vi "serial cmd-response.vi"(0 "VISA In":refnum<visa-resource-name>, 1 "mode":enum16{"wr & rd", "write", "read"}(ring), 3 "flush transcvr(F)":bool, 5 "cmd":string, 9 "ReadWait":u32=50, 11 "error in":errorcluster, 12 "Sem Timeout (5000)":i32=5000) -> (4 "VISA out":refnum<visa-resource-name>, 6 "rsp str out":string, 8 "cmd str out":string, 10 "timeout?":bool, 15 "error out":errorcluster)   [LabVIEW 2017]
doc: "Developed by: Kevin Thompson\nThompson Engineering\nthompson.engineering@comcast.net\n(510) 673-3614"
uses:
  <vilib>/Instr/_visa.llb/VISA Flush IO Buffer Mask.ctl
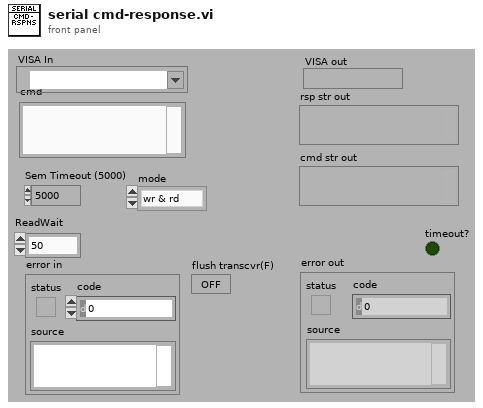
[diagram p1: front panel]
types:
  T1 = typedef "Semaphore RefNum" = refnum<k1>
  T2 = typedef "VISA Flush IO Buffer Mask.ctl" = u16
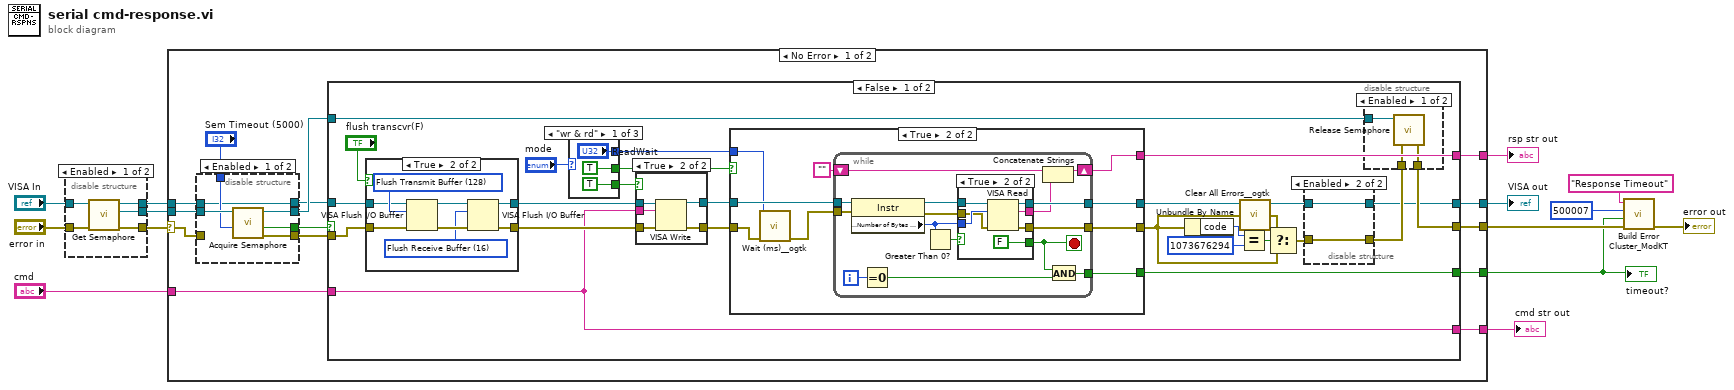
[diagram p0: block diagram]
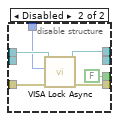
[diagram p3: hidden frame]
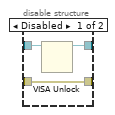
[diagram p4: hidden frame]
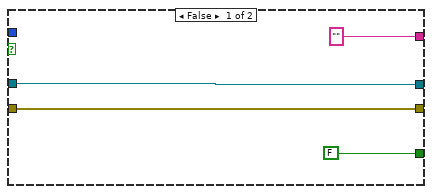
[diagram p7: hidden frame]
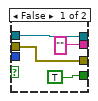
[diagram p8: hidden frame]
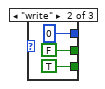
[diagram p10: hidden frame]
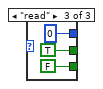
[diagram p11: hidden frame]
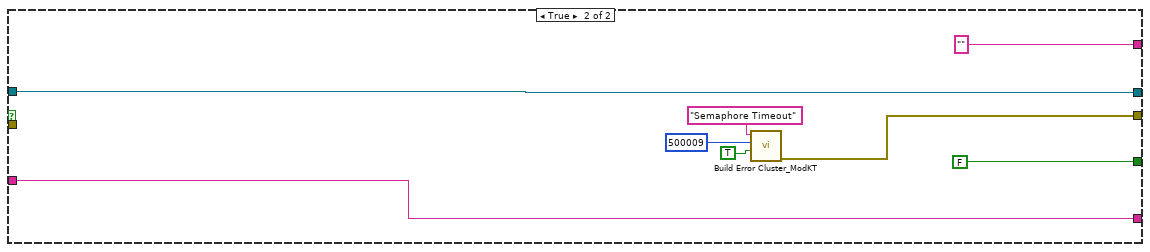
[diagram p12: hidden frame]
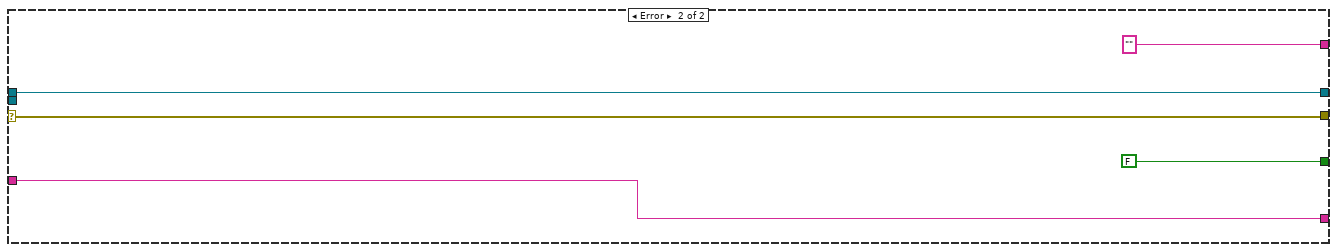
[diagram p13: hidden frame]
diagram:
  n1 = disable-structure shown="Enabled" {
    disable-tunnel: "VISA In" -> [w19 w21]
    disable-tunnel: "error in" -> [w18 w20]
    disable-tunnel: [w17 w21] -> w6
    disable-tunnel: [w16 w20] -> w5
    disable-tunnel: [w15 _] -> w4
    frame Enabled {
      n2 = call "Get Semaphore.vi"("error in"=w18, "VISA In"=w19) -> ("error out"=w16:errorcluster, "semaphore out"=w15:T1, "VISA Out"=w17:refnum<visa-resource-name>)  [unwired: 3 in]
    }
    frame Disabled {
    }
  }
  n3 = case shown="No Error" w5 {
    selector: w5 -> [w22 w156]
    tunnel: [w35 FALSE] -> w11
    tunnel: [w34 "" ("read buffer")] -> w14
    tunnel: w6 -> [w24 w157]
    tunnel: [w33 w157] -> w13
    tunnel: [w32 w156] -> w12
    tunnel: w4 -> [w31 _]
    tunnel: "cmd" -> [w26 w155]
    tunnel: [w25 w155] -> w2
    frame No Error {
      n4 = disable-structure shown="Enabled" {
        disable-tunnel: w31 -> [w41 _]
        disable-tunnel: "Sem Timeout (5000)" -> [w40 w42]
        disable-tunnel: [w39 FALSE ("timed out")] -> w29
        disable-tunnel: [w38 _] -> w28
        disable-tunnel: [w37 w47] -> w27
        disable-tunnel: w24 -> [w36 w46]
        disable-tunnel: [w36 w45] -> w23
        disable-tunnel: w22 -> [_ w44]
        frame Enabled {
          n5 = call <vilib>:"Acquire Semaphore.vi"("ms timeout (-1)"=w40, "semaphore"=w41) -> ("error out"=w37:errorcluster, "timed out"=w39:bool, "semaphore out"=w38:T1)  [unwired: 3 in]
        }
        frame Disabled {
          n6 = call <vilib>:"VISA Lock Async.vi"("error in (no error)"=w44, "timeout (0)"=w42, "VISA resource name"=w46) -> ("error out"=w47:errorcluster, "VISA resource name out"=w45:refnum<visa-resource-name>)  [unwired: 6 in, 1 out]
        }
      }
      n7 = case shown="False" w29 {
        tunnel: [w63 "" ("read buffer")] -> w34
        tunnel: [w62 FALSE] -> w35
        tunnel: w23 -> [w61 w152]
        tunnel: [w56 w149] -> w32
        tunnel: [w48 w152] -> w33
        tunnel: w28 -> [w57 _]
        tunnel: w27 -> [w55 _]
        tunnel: w26 -> [w54 w147]
        tunnel: [w54 w147] -> w25
        frame False {
          n8 = case shown="True" "flush transcvr(F)" {
            tunnel: w61 -> [w83 w90]
            tunnel: [w82 w87] -> w60
            tunnel: [w83 w86] -> w59
            tunnel: w55 -> [w82 w84]
            frame False {
            }
            frame True {
              w85 = T2 16 items=["Flush Receive Buffer"=16, "Write Transmit Buffer to Device"=32, "Flush Receive Buffer (No I/O)"=64, "Flush Transmit Buffer"=128] ("Mask")
              w91 = T2 128 items=["Flush Receive Buffer"=16, "Write Transmit Buffer to Device"=32, "Flush Receive Buffer (No I/O)"=64, "Flush Transmit Buffer"=128] ("Mask")
              n9 = VISA Flush I/O Buffer(VISA resource name=w90, mask (16)=w91, error in (no error)=w84) -> (VISA resource name out=w88:refnum<visa-resource-name>, error out=w89:errorcluster)
              n10 = VISA Flush I/O Buffer(VISA resource name=w88, mask (16)=w85, error in (no error)=w89) -> (VISA resource name out=w86:refnum<visa-resource-name>, error out=w87:errorcluster)
            }
          }
          n11 = case shown="\"wr & rd\"" "mode" {
            tunnel: [TRUE TRUE FALSE] -> w70
            tunnel: [TRUE FALSE TRUE] -> w69
            tunnel: ["ReadWait" u32 0 ("wait (ms)") u32 0 ("wait (ms)")] -> w53
            frame "wr & rd" {
            }
            frame "write" {
            }
            frame "read" {
            }
          }
          n12 = case shown="True" w70 {
            tunnel: [w132 w137] -> w72
            tunnel: [w131 w136] -> w52
            tunnel: w59 -> [w132 w135]
            tunnel: w54 -> [_ w134]
            tunnel: w60 -> [w131 w133]
            frame False {
            }
            frame True {
              n13 = VISA Write(VISA resource name=w135, write buffer=w134, error in (no error)=w133) -> (VISA resource name out=w137:refnum<visa-resource-name>, error out=w136:errorcluster)  [unwired: 1 out]
            }
          }
          n14 = case shown="True" w69 {
            tunnel: w72 -> [w93 w104]
            tunnel: [FALSE w100] -> w62
            tunnel: [w93 w103] -> w49
            tunnel: ["" ("read buffer") w99] -> w63
            tunnel: [w92 w102] -> w64
            tunnel: w53 -> [_ w98]
            tunnel: w52 -> [w92 w97]
            frame False {
            }
            frame True {
              n15 = call <userlib>:"Wait (ms)__ogtk.vi"("error in (no error)"=w97, "milliseconds to wait"=w98) -> ("error out"=w96:errorcluster)  [unwired: 8 in, 1 out]
              n16 = while {
                tunnel: w104 -> [w119]
                tunnel: w96 -> [w114]
                tunnel: [w113] -> w103
                tunnel: [w112] -> w102
                shift-right: [w109] -> w99
                shift-left: "" -> [w111]
                tunnel: [w105] -> w100
                i -> [w107]
                stop <- w108 stop-if-true
                n17 = property class="Instr"(reference=w119, error in=w114) -> (reference out=w116:refnum<visa-resource-name>, error out=w117:errorcluster, "Serial Settings:Number of Bytes at Serial Port"=w115:u32)
                n18 = Equal To 0?(x=w107) -> (x = 0?=w106:bool)
                n19 = Greater Than 0?(x=w115) -> (x > 0?=w118:bool)
                n20 = case shown="True" w118 {
                  tunnel: w115 -> [_ w130]
                  tunnel: w116 -> [w121 w124]
                  tunnel: w117 -> [w122 w129]
                  tunnel: [TRUE FALSE] -> w108
                  tunnel: ["" ("read buffer") w127] -> w110
                  tunnel: [w122 w126] -> w112
                  tunnel: [w121 w125] -> w113
                  frame False {
                  }
                  frame True {
                    n21 = VISA Read(VISA resource name=w124, byte count=w130, error in (no error)=w129) -> (VISA resource name out=w125:refnum<visa-resource-name>, read buffer=w127:string, error out=w126:errorcluster)  [unwired: 1 out]
                  }
                }
                n22 = Concatenate Strings(w111, w110) -> (w109:string)
                n23 = And(x=w108, y=w106) -> (x .and. y?=w105:bool)
              }
            }
          }
          n24 = Unbundle By Name(w64) -> ("code"=w68:i32)
          n25 = Equal?(x=w68, y=1073676294 ("error code")) -> (x = y?=w66:bool)
          n26 = call <userlib>:"Clear All Errors__ogtk.vi"("Error In"=w64) -> ("Error Out"=w65:errorcluster)  [unwired: 3 in]
          n27 = Select(t=w65, s=w66, f=w64) -> (s? t:f=w51:errorcluster)
          n28 = disable-structure shown="Enabled" {
            disable-tunnel: w51 -> [w73 w76]
            disable-tunnel: [w73 w76] -> w50
            disable-tunnel: w49 -> [w75 w77]
            disable-tunnel: [w74 w77] -> w48
            frame Disabled {
              n29 = VISA Unlock(11:w75) -> (3:w74:refnum<visa-resource-name>)  [unwired: 1 in, 1 out]
            }
            frame Enabled {
            }
          }
          n30 = disable-structure shown="Enabled" {
            disable-tunnel: w57 -> [w80 _]
            disable-tunnel: w50 -> [w79 w81]
            disable-tunnel: [w78 w81] -> w56
            frame Enabled {
              n31 = call <vilib>:"Release Semaphore.vi"("error in (no error)"=w79, "semaphore"=w80) -> ("error out"=w78:errorcluster)  [unwired: 4 in, 1 out]
            }
            frame Disabled {
            }
          }
        }
        frame True {
          n32 = call <vilib>:"Build Error Cluster_ModKT .vi"("Prepend String (\"\")"="Semaphore Timeout" ("Prepend String (\"\")"), "code"=500009, "error? (F)"=TRUE) -> ("error out"=w149:errorcluster)  [unwired: 4 in, 1 out]
        }
      }
    }
    frame Error {
    }
  }
  "timeout?" <- w11
  "rsp str out" <- w14
  "VISA out" <- w13
  "cmd str out" <- w2
  n33 = call <vilib>:"Build Error Cluster_ModKT .vi"("Prepend String (\"\")"="Response Timeout" ("Prepend String (\"\")"), "code"=500007, "error? (F)"=w11, "error in (no error)"=w12) -> ("error out"=→"error out":errorcluster)  [unwired: 3 in, 1 out]
